vi "Zero.vi"(8 "error in":errorcluster, 11 "Neph in":refnum<class "Nephelometer.lvclass">) -> (0 "error out":errorcluster, 3 "Neph out":refnum<class "Nephelometer.lvclass">)   [LabVIEW 2014, in "Nephelometer.lvclass"]
uses:
  Nephelometer.lvclass
  Reusable/Session APIs/Serial/Serial Session.lvclass
  Nephelometer.lvclass/Nephelometer.ctl
  Reusable/Session APIs/Text Communication/Text Device Session.lvclass/Text Device Session.ctl
  Accessors/Read Session Handle.vi
  Reusable/Session APIs/Text Communication/Read hSysLog.vi
  <userlib>/_Session Fwk/Session - Root.lvclass
  Reusable/Session Log/System Log.lvclass
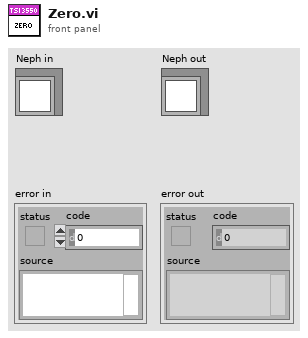
[diagram p1: front panel]
types:
  T1 = typedef "Session - Root.lvclass/Session Handle.ctl" = refnum<data-value>
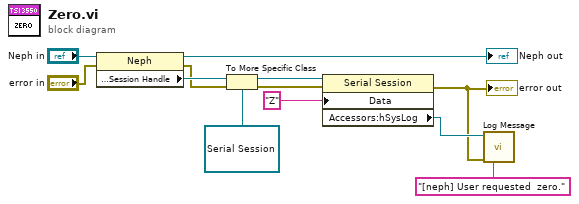
[diagram p0: block diagram]
diagram:
  n1 = property class="Neph"(reference="Neph in", error in="error in") -> (reference out=→"Neph out":refnum<class "Nephelometer.lvclass">, error out=w2:errorcluster, "Accessors:Session Handle"=w7:T1)
  n2 = To More Specific Class(target class=refnum<data-value> refnum ("Session Handle"), reference=w7, error in=w2) -> (specific class reference=w6:refnum<data-value>, error out=w1:errorcluster)
  n3 = property class="Serial Session"(reference=w6, error in=w1, "Data"="Z" ("Write - Asynchronous")) -> (error out=w3:errorcluster, "Accessors:hSysLog"=w5:T1)  [unwired: 1 out]
  "error out" <- w3
  n4 = call "Log Message.vi"("error in"=w3, "MSG In"="[neph] User requested  zero.", "session in"=w5) -> ()  [unwired: 7 in, 2 out]
